vi "GetWave-DPO4000.vi"(2 "Channel":u8(ring) caption="Select Waveform" items=["Channel 1", "Channel 2", "Channel 3", "Channel 4", "Math", "Reference 1", "Reference 2", "Reference 3", "Reference 4"], 3 "Data Width":u8(ring) items=["1", "2"], 4 "Scope":refnum<visa-resource-name>) -> (8 "Waveform Array":dbl[](array[numeric]))   [LabVIEW 2014]
doc: "Get waveform data array from the specified input channel on the Tektronix DPO 4XXX scope. Consists of 8-bit values ranging from 0-255."
panel:
  out "error out":errorcluster
  out "Bytes Read":i32
  out "Array Elements":i32
  out "Points Read":dbl
  # "Tektronix DPO 4000 Digital Oscillocope Series"
  # "Input Parameters"
  # "Output Parameters"
  # "This program retrieves the waveform data in an array \nfrom the specified channel.\n\nData Structure\n#<L><Data Points><Data><If>\n\n<Data Points>: number of elements in the data array\n<L>:  the number of digits in <DataPoints>\n\nNote: Total bytes read depends on value of data width.\nDefaults:  DATA:WIDTH1     DATA:ENCDG RPBNARY\n\nhttp://www.tek.com/product-support-hub/mso4000-dpo4000"
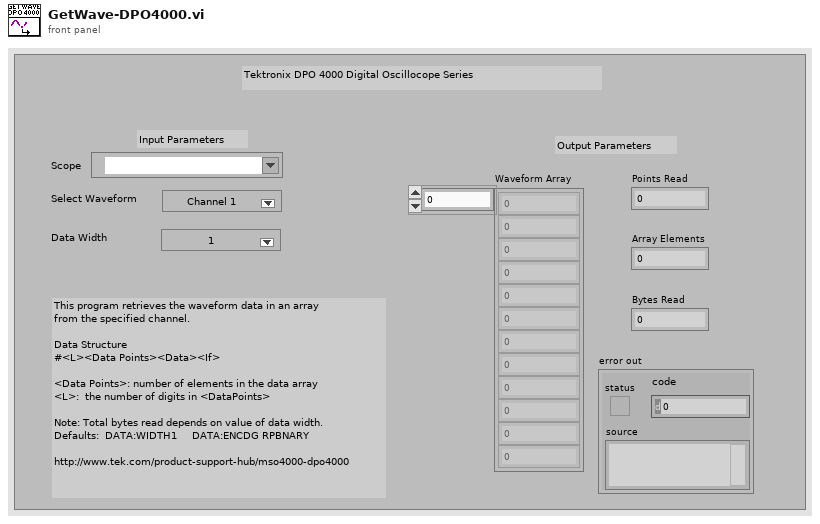
[diagram p1: front panel]
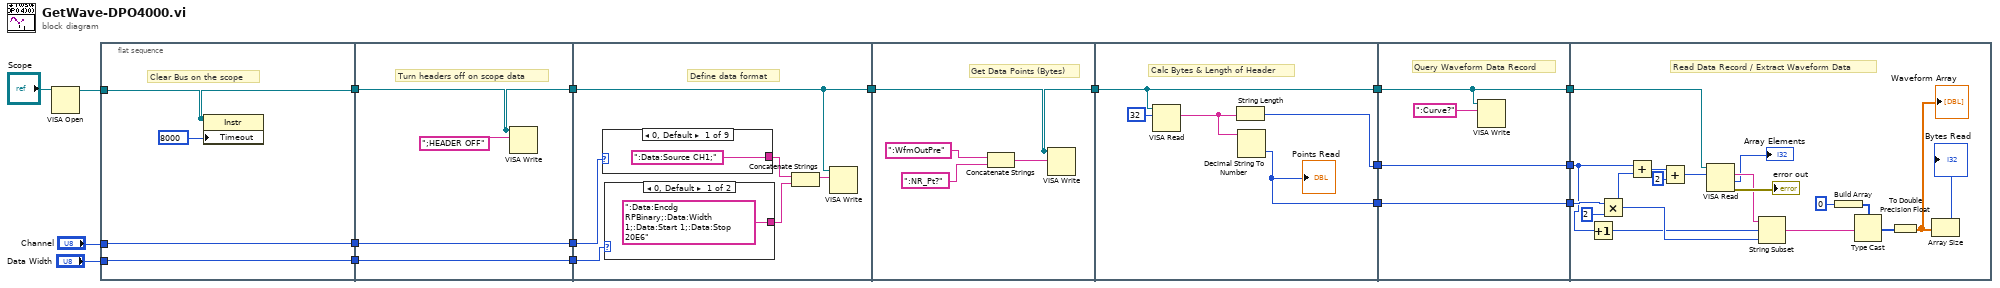
[diagram p0: block diagram]
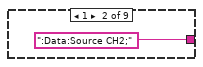
[diagram p2: hidden frame]
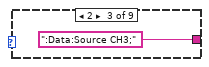
[diagram p3: hidden frame]
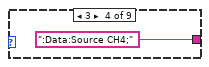
[diagram p4: hidden frame]
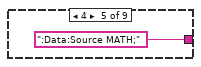
[diagram p5: hidden frame]
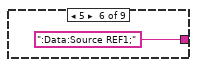
[diagram p6: hidden frame]
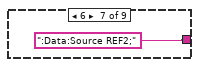
[diagram p7: hidden frame]
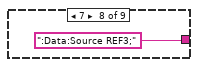
[diagram p8: hidden frame]
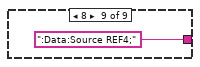
[diagram p9: hidden frame]
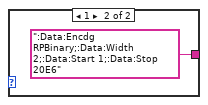
[diagram p10: hidden frame]
diagram:
  n1 = VISA Open(VISA resource name="Scope") -> (VISA resource name=w1:refnum<visa-resource-name>)  [unwired: 4 in, 1 out]
  n2 = flat-sequence {
    tunnel: w1 -> [w21]
    tunnel: "Data Width" -> [w20]
    tunnel: "Channel" -> [w19]
    tunnel: [w21] -> w16
    tunnel: [w20] -> w15
    tunnel: [w19] -> w14
    tunnel: w16 -> [w25]
    tunnel: w15 -> [w24]
    tunnel: w14 -> [w23]
    tunnel: [w25] -> w13
    tunnel: [w24] -> w12
    tunnel: [w23] -> w11
    tunnel: w13 -> [w27]
    tunnel: w12 -> [w28]
    tunnel: w11 -> [w29]
    tunnel: [w27] -> w10
    tunnel: w10 -> [w44]
    tunnel: [w44] -> w9
    tunnel: w9 -> [w52]
    tunnel: [w52] -> w8
    tunnel: [w49] -> w7
    tunnel: [w48] -> w6
    tunnel: w8 -> [w55]
    tunnel: w7 -> [w53]
    tunnel: w6 -> [w54]
    tunnel: [w55] -> w5
    tunnel: [w54] -> w4
    tunnel: [w53] -> w3
    tunnel: w5 -> [w74]
    tunnel: w4 -> [w73]
    tunnel: w3 -> [w66]
    frame #0 {
      # "Clear Bus on the scope"
      n3 = property class="Instr"(reference=w21, "Timeout"=u32 8000 ("General Settings:Timeout Value")) -> ()  [unwired: 1 in, 2 out]
    }
    frame #1 {
      # "Turn headers off on scope data"
      n4 = VISA Write(VISA resource name=w25, write buffer=";HEADER OFF") -> ()  [unwired: 1 in, 3 out]
    }
    frame #2 {
      # "Define data format"
      n5 = case shown="0, Default" w29 {
        tunnel: [":Data:Source CH1;" ":Data:Source CH2;" ":Data:Source CH3;" ":Data:Source CH4;" ":Data:Source MATH;" ":Data:Source REF1;" ":Data:Source REF2;" ":Data:Source REF3;" ":Data:Source REF4;"] -> w32
        frame 0, Default {
        }
        frame 1 {
        }
        frame 2 {
        }
        frame 3 {
        }
        frame 4 {
        }
        frame 5 {
        }
        frame 6 {
        }
        frame 7 {
        }
        frame 8 {
        }
      }
      n6 = case shown="0, Default" w28 {
        tunnel: [":Data:Encdg RPBinary;:Data:Width 1;:Data:Start 1;:Data:Stop 20E6" ":Data:Encdg RPBinary;:Data:Width 2;:Data:Start 1;:Data:Stop 20E6"] -> w31
        frame 0, Default {
        }
        frame 1 {
        }
      }
      n7 = Concatenate Strings(w32, w31) -> (w30:string)
      n8 = VISA Write(VISA resource name=w27, write buffer=w30) -> ()  [unwired: 1 in, 3 out]
    }
    frame #3 {
      # "Get Data Points (Bytes)"
      n9 = Concatenate Strings(":WfmOutPre", ":NR_Pt?") -> (w45:string)
      n10 = VISA Write(VISA resource name=w44, write buffer=w45) -> ()  [unwired: 1 in, 3 out]
    }
    frame #4 {
      # "Calc Bytes & Length of Header"
      n11 = VISA Read(VISA resource name=w52, byte count=u32 32) -> (read buffer=w50:string)  [unwired: 1 in, 3 out]
      n12 = String Length(string=w50) -> (length=w49:i32)
      n13 = Decimal String To Number(string=w50) -> (number=w48:i32)  [unwired: 2 in, 1 out]
      "Points Read" <- w48
    }
    frame #5 {
      # "Query Waveform Data Record"
      n14 = VISA Write(VISA resource name=w55, write buffer=":Curve?") -> ()  [unwired: 1 in, 3 out]
    }
    frame #6 {
      # "Read Data Record / Extract Waveform Data"
      n15 = Increment(x=w66) -> (x+1=w65:i32)
      n16 = Multiply(x=w73, y=2) -> (x*y=w67:i32)
      n17 = Add(x=w66, y=w67) -> (x+y=w72:i32)
      n18 = Add(x=w72, y=2) -> (x+y=w70:i32)
      n19 = VISA Read(VISA resource name=w74, byte count=w70) -> (read buffer=w68:string, return count=→"Array Elements":u32, error out=→"error out":errorcluster)  [unwired: 1 in, 1 out]
      n20 = String Subset(string=w68, offset (0)=w65, length (rest)=w67) -> (substring=w62:string)
      n21 = Build Array ("U8 Array Type")(u8 0 ("element")) -> (w60:u8[])
      n22 = Type Cast ("Byte Count")(type=w60, x=w62) -> (*(type *) &x=w59:u8[])
      n23 = To Double Precision Float(number=w59) -> (double precision float=w57:dbl[])
      "Waveform Array" <- w57
      n24 = Array Size(array=w57) -> (size(s)=→"Bytes Read":i32)
    }
  }
